vi "Riffle Array (CDB) (obs 2012).vi"(10 "seed":i32=-1, 11 "X":cdb[](array[numeric])) -> (0 "error":i32, 2 "Riffled Index":i32[](array[numeric]), 3 "Riffled {X}":cdb[](array[numeric]))   [LabVIEW 2017, in "NI_AALBase.lvlib"]
doc: "Riffles the elements in the input array <B>X</B>. Wire data to the <B>X</B> input to determine the polymorphic instance to use or manually select the instance."
uses:
  NI_AALBase.lvlib
  lvanlys.dll
panel:
  # "Riffle Array (CDB)"
  # "This VI is obsolete !!!\nYou should replace this VI in your diagram with the Riffle VI."
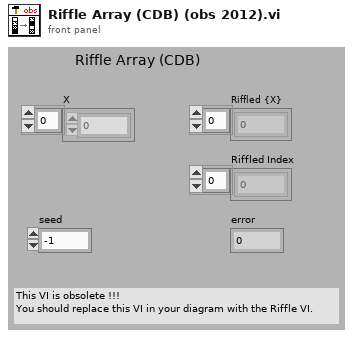
[diagram p1: front panel]
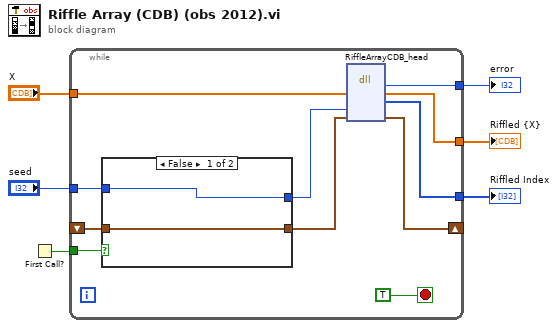
[diagram p0: block diagram]
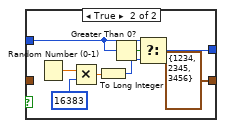
[diagram p2: hidden frame]
diagram:
  n1 = First Call?() -> (First Call?: T/F=w6:bool)
  n2 = while {
    tunnel: "seed" -> [w16]
    shift-right: [w9] -> _
    shift-left: _ -> [w14]
    tunnel: w6 -> [w15]
    tunnel: [w13] -> w3
    tunnel: [w12] -> w5
    tunnel: "X" -> [w11]
    tunnel: [w7] -> w1
    stop <- TRUE stop-if-true
    n3 = case shown="False" w15 {
      tunnel: w14 -> [w19 _]
      tunnel: [w19 cluster{"xSeed":i32, "ySeed":i32, "zSeed":i32} {"xSeed"=1234, "ySeed"=2345, "zSeed"=3456} ("RNGState")] -> w10
      tunnel: [w18 w25] -> w8
      tunnel: w16 -> [w18 w26]
      frame False {
      }
      frame True {
        n4 = Random Number (0-1)() -> (number: 0 to 1=w23:dbl)
        n5 = Multiply(x=w23, y=16383 ("x")) -> (x*y=w24:dbl)
        n6 = To Long Integer(number=w24) -> (32bit integer=w22:i32)
        n7 = Greater Than 0?(x=w26) -> (x > 0?=w27:bool)
        n8 = Select(t=w26, s=w27, f=w22) -> (s? t:f=w25:i32)
      }
    }
    n9 = dll-call lib="C:/Program Files/National Instruments/LabVIEW 2017/resource/lvanlys.*" fn="RiffleArrayCDB_head"("X"=w11, "seed"=w8, "RNGState"=w10) -> (w13:i32, "X"=w12:cdb[], "riffleIndex"=w7:i32[], "RNGState"=w9:cluster{"xSeed":i32, "ySeed":i32, "zSeed":i32})  [unwired: 5 in, 2 out]
  }
  "Riffled {X}" <- w5
  "error" <- w3
  "Riffled Index" <- w1
